vi "estimate detection parameters.vi"(1 "PMT for triggering":i32, 7 "Sorting Timetrace":cluster{dbl, dbl, dbl[][]}) -> (4 "peak max":dbl, 6 "peak min":dbl, 8 "max duration":dbl, 10 "min duration":dbl)   [LabVIEW 2009]
uses:
  <vilib>/Analysis/2dsp.llb/Real FFT.vi
  <vilib>/Analysis/NI_AALPro.lvlib
panel:
  out "time trace":dbl[](graph)
  out "powerspectrum":dbl[](graph)
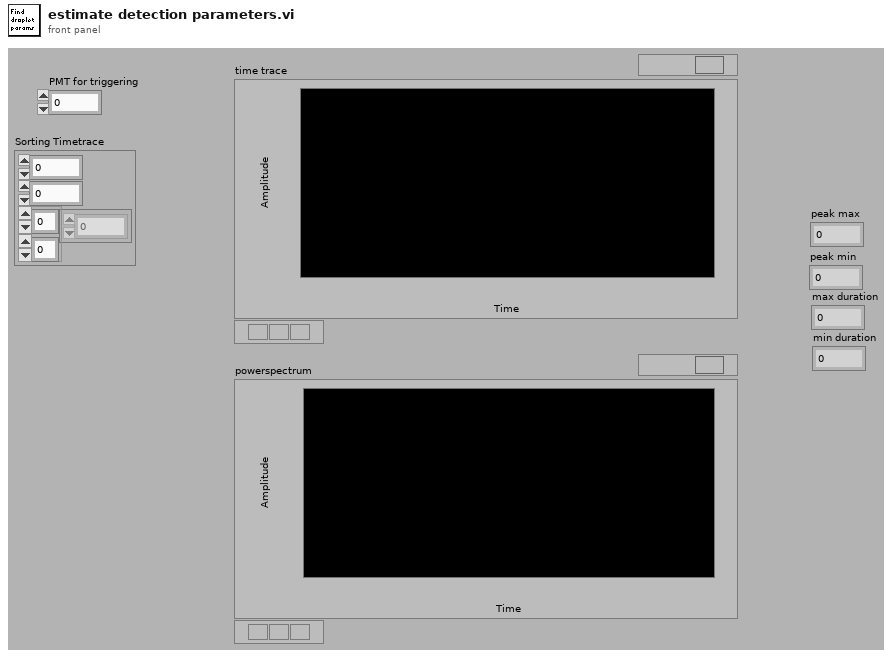
[diagram p1: front panel]
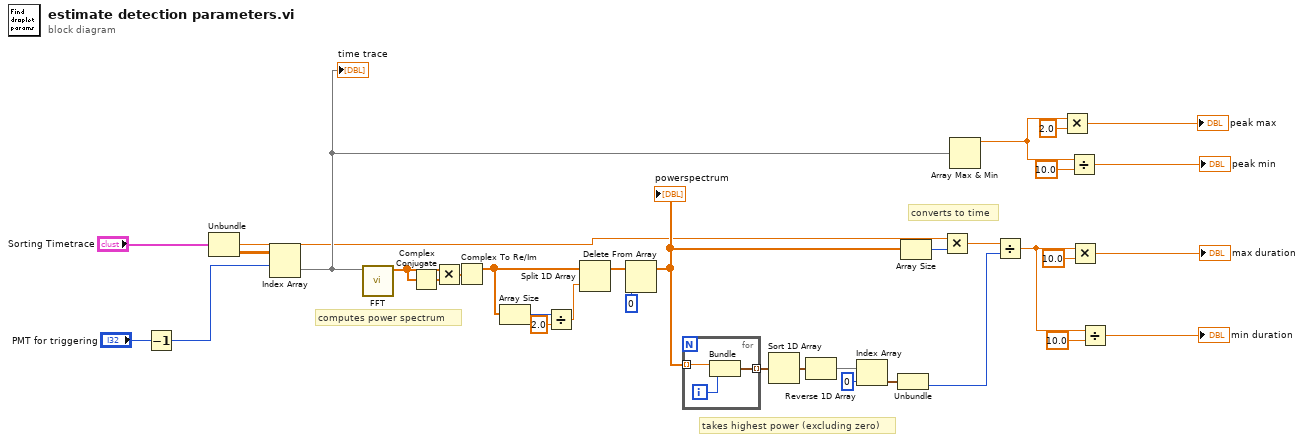
[diagram p0: block diagram]
diagram:
  # "converts to time"
  # "takes highest power (excluding zero)"
  # "computes power spectrum"
  n1 = Decrement(x="PMT for triggering") -> (x-1=w6:i32)
  n2 = Unbundle("Sorting Timetrace") -> (w2:dbl, w31:dbl[][])  [unwired: 1 out]
  n3 = Index Array(array=w31, index (row)=w6) -> (element=w5:dbl[])  [unwired: 1 in]
  "time trace" <- w5
  n4 = call-poly <vilib>:"FFT.vi"("X"=w5) -> ("FFT {X}"=w30:cdb[])  [unwired: 9 in, 1 out]
  n5 = Complex Conjugate(1:w30) -> (0:w29:cdb[])
  n6 = Multiply(x=w30, y=w29) -> (x*y=w28:cdb[])
  n7 = Complex To Re/Im(x + iy=w28) -> (x=w11:dbl[])  [unwired: 1 out]
  n8 = Array Size(array=w11) -> (size(s)=w13:i32)
  n9 = Divide(x=w13, y=2.0) -> (x/y=w12:dbl)
  n10 = Split 1D Array(array=w11, index=w12) -> (first subarray=w9:dbl[])  [unwired: 1 out]
  n11 = Delete From Array(array=w9, index=0) -> (array with subset deleted=w8:dbl[])  [unwired: 1 in, 1 out]
  "powerspectrum" <- w8
  n12 = for {
    tunnel: w8 -> [w37] mode=indexing
    tunnel: [w35] -> w27 mode=indexing
    i -> [w36]
    n13 = Bundle(w37, w36) -> (w35:cluster{dbl, i32})  [unwired: 1 in]
  }
  n14 = Sort 1D Array(array=w27) -> (sorted array=w26:cluster{dbl, i32}[])
  n15 = Reverse 1D Array(array=w26) -> (reversed array=w7:cluster{dbl, i32}[])
  n16 = Index Array(array=w7, index=0) -> (element=w24:cluster{dbl, i32})
  n17 = Unbundle(w24) -> (w21:i32)  [unwired: 1 out]
  n18 = Array Size(array=w8) -> (size(s)=w23:i32)
  n19 = Multiply(x=w2, y=w23) -> (x*y=w22:dbl)
  n20 = Array Max & Min(array=w5) -> (max value=w15:dbl)  [unwired: 3 out]
  n21 = Divide(x=w22, y=w21) -> (x/y=w20:dbl)
  n22 = Multiply(x=w15, y=2.0) -> (x*y=→"peak max":dbl)
  n23 = Divide(x=w15, y=10.0) -> (x/y=→"peak min":dbl)
  n24 = Multiply(x=w20, y=10.0) -> (x*y=→"max duration":dbl)
  n25 = Divide(x=w20, y=10.0) -> (x/y=→"min duration":dbl)
